vi "Communicate - Initialize.vi"(8 "error in (no error)":errorcluster, 11 "Generator/Remote Config":path) -> (0 "error out":errorcluster, 1 "Write Queue(s)":refnum<queue>[](array[refnum]), 2 "Read Queue(s)":refnum<queue>[](array[refnum]), 3 "TCP Connection ID(s)":refnum<k5>[](array[refnum]))   [LabVIEW 2020]
doc: "Author: Erich Schlieper\n\nTakes the input of the <B>Generator/Remote Config</B> file and reads that config file looking for TCP/IP addresses for which communication ports should be opened and queues will be created to manage potentially multiple TCP sessions. A read and write queue is created for each TCP/IP session so that specific messages can be sent to specific generators or remote units based on the application."
uses:
  <vilib>/Utility/config.llb/Read Key (String).vi
  <vilib>/Utility/config.llb/NI_LVConfig.lvlib
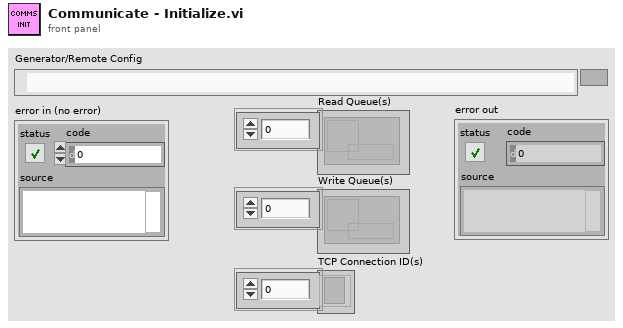
[diagram p1: front panel]
types:
  T1 = typedef "NI_LVConfig.lvlib/Config Data RefNum.ctl" = refnum<k1>
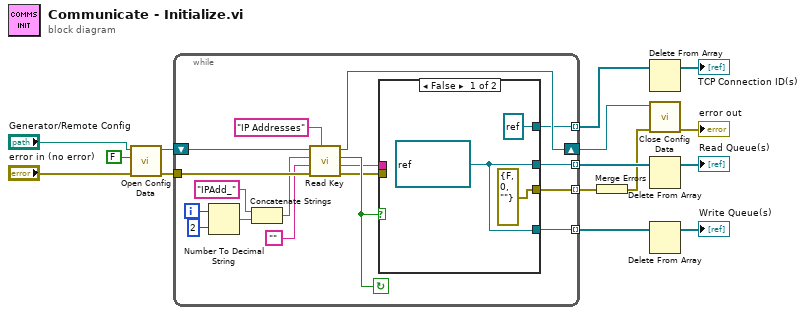
[diagram p0: block diagram]
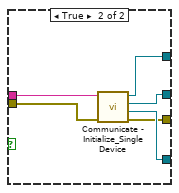
[diagram p2: hidden frame]
diagram:
  n1 = call <vilib>:"Open Config Data.vi"("error in (no error)"="error in (no error)", "create file if necessary (T)"=FALSE, "configuration file path"="Generator/Remote Config") -> ("error out"=w11:errorcluster, "refnum"=w12:T1)  [unwired: 6 in, 1 out]
  n2 = while {
    tunnel: w11 -> [w31]
    shift-right: [w20] -> w7
    shift-left: w12 -> [w32]
    tunnel: [w19] -> w9 mode=indexing
    tunnel: [w18] -> w10 mode=indexing
    tunnel: [w17] -> w8 mode=indexing
    tunnel: [w16] -> w2 mode=indexing
    i -> [w27]
    stop <- w23 continue-if-true
    n3 = Number To Decimal String(number=w27, width (-)=i16 2) -> (decimal integer string=w28:string)
    n4 = Concatenate Strings("IPAdd_" ("section"), w28) -> (w25:string)
    n5 = call-poly <vilib>:"Read Key.vi"("section"="IP Addresses", "error in (no error)"=w31, "default value"="", "key"=w25, "refnum"=w32) -> ("error out"=w21:errorcluster, "value"=w22:string, "found?"=w23:bool, "refnum out"=w20:T1)  [unwired: 3 in]
    n6 = case shown="False" w23 {
      tunnel: w22 -> [_ w41]
      tunnel: w21 -> [_ w40]
      tunnel: [w34 w39] -> w19
      tunnel: [w34 w38] -> w18
      tunnel: [errorcluster {"status"=FALSE, "code"=0, "source"=""} ("error IO") w37] -> w17
      tunnel: [refnum<k5> refnum ("connection ID") w36] -> w16
      frame False {
        w34 = refnum<queue> refnum ("queue out")
      }
      frame True {
        n7 = call "Communicate - Initialize_Single Device.vi"("error in (no error)"=w40, "IP Address"=w41) -> ("error out"=w37:errorcluster, "Write Queue Out"=w39:refnum<queue>, "Read Queue Out"=w38:refnum<queue>, "TCP Network Connection out"=w36:refnum<k5>)  [unwired: 6 in]
      }
    }
  }
  n8 = Merge Errors(w8) -> (w6:errorcluster)
  n9 = Delete From Array(array=w2) -> (array with subset deleted=→"TCP Connection ID(s)":refnum<k5>[])  [unwired: 2 in, 1 out]
  n10 = call <vilib>:"Close Config Data.vi"("error in (no error)"=w6, "refnum"=w7) -> ("error out"=→"error out":errorcluster)  [unwired: 8 in, 1 out]
  n11 = Delete From Array(array=w10) -> (array with subset deleted=→"Read Queue(s)":refnum<queue>[])  [unwired: 2 in, 1 out]
  n12 = Delete From Array(array=w9) -> (array with subset deleted=→"Write Queue(s)":refnum<queue>[])  [unwired: 2 in, 1 out]
